vi "Write Channel Setting.vi"(8 "error in (no error)":errorcluster, 10 "Channel Settings":T1={"Amplitude"=0.0, "Vertical Coupling"=enum."DC", "Probe Attenuation"=0.0, "Enable?"=FALSE, "Maximum Input Frequency"=0.0, "Input Impedance"=0, "Timeout (s)"=5.0} {"Timeout (s)" format="%.2f"; "Input Impedance" items=["1 mega ohm", "50 ohms"]; "Maximum Input Frequency" format="%.2f"}, 11 "Oscilloscope in":refnum<class "Oscilloscope.lvclass">) -> (0 "error out":errorcluster, 3 "Oscilloscope out":refnum<class "Oscilloscope.lvclass">)   [LabVIEW 2019, in "Oscilloscope.lvlib" / "Oscilloscope.lvclass"]
uses:
  Oscilloscope.lvclass
  Custom Controls/Channel Settings.ctl
  Custom Controls/Vertical Coupling.ctl
  Oscilloscope.lvclass/Oscilloscope.ctl
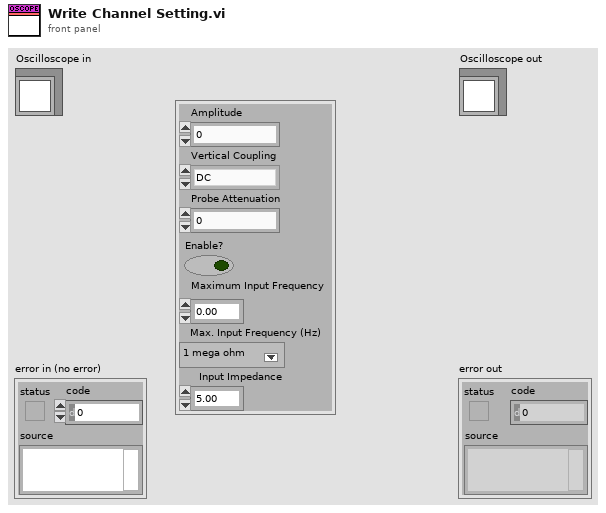
[diagram p1: front panel]
types:
  T1 = typedef "Oscilloscope.lvlib/Oscilloscope.lvclass/Channel Settings.ctl" = cluster{"Amplitude":dbl, "Vertical Coupling":T2, "Probe Attenuation":dbl, "Enable?":bool, "Maximum Input Frequency":dbl, "Input Impedance":u16, "Timeout (s)":dbl}
  T2 = typedef "Oscilloscope.lvlib/Oscilloscope.lvclass/Vertical Coupling.ctl" = enum16{"AC", "DC", "Ground"}
  T3 = typedef "Oscilloscope.lvlib/Oscilloscope.lvclass/Channel List.ctl" = u16
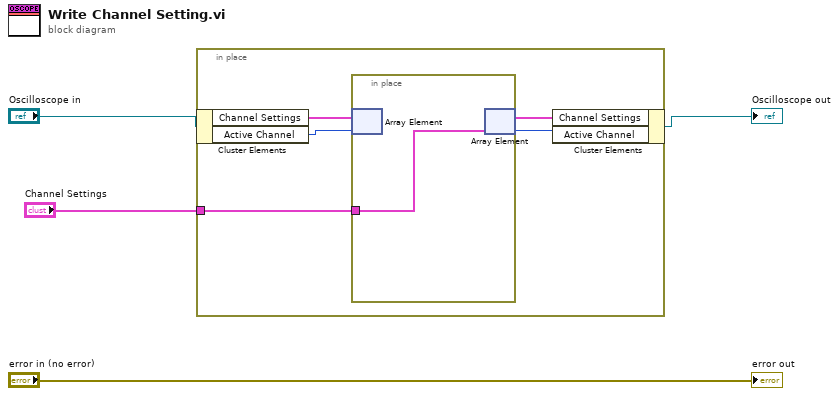
[diagram p0: block diagram]
diagram:
  n1 = in-place {
    in-place-border: "Channel Settings" -> [w5]
    n2 = in-place-cluster #1("Oscilloscope in") -> ("Channel Settings"=w9:T1[], "Active Channel"=w7:T3)
    n3 = in-place {
      in-place-border: w5 -> [w10]
      n4 = in-place-array #2(w9, w7) -> ()  [unwired: 1 out]
      n5 = in-place-array #2(w10) -> (w8:T1[], w6:i32)
    }
    n6 = in-place-cluster #1("Channel Settings"=w8, "Active Channel"=w6) -> (→"Oscilloscope out":refnum<class "Oscilloscope.lvclass">)
  }
  "error out" <- "error in (no error)"
